vi "Register Sensor View.vi"(11 "Message Enqueuer in":refnum<class "Message Enqueuer.lvclass">) -> (3 "Message Enqueuer out":refnum<class "Message Enqueuer.lvclass">)   [LabVIEW 2013]
uses:
  <vilib>/ActorFramework/Message Enqueuer/Message Enqueuer.lvclass
  <vilib>/ActorFrameworkMVC/View Observer/Registration Message/Registration Message.lvclass
  <vilib>/ActorFrameworkMVC/View Observer/Data Message/Data Message.lvclass
  Models/Sensor Model Messages/Register Sensor Tiles Info Msg/Register Sensor Tiles Info Msg.lvclass
  Models/Sensor Model Messages/Register Sensor Previous Button Visibility Msg/Register Sensor Previous Button Visibility Msg.lvclass
  Models/Sensor Model Messages/Register Sensor Next Button Visibility Msg/Register Sensor Next Button Visibility Msg.lvclass
  Views/Sensor View Messages/Conceret Sensor Tiles Info Msg/Conceret Sensor Tiles Info Msg.lvclass
  Views/Sensor View Messages/Conceret Sensor Previous Button Visibility Msg/Conceret Sensor Previous Button Visibility Msg.lvclass
  Views/Sensor View Messages/Conceret Sensor Next Button Visibility Msg/Conceret Sensor Next Button Visibility Msg.lvclass
  Models/Sensor Model Messages/Register Sensor Move In Previous Msg/Register Sensor Move In Previous Msg.lvclass
  Views/Sensor View Messages/Conceret Move In Previous Msg/Conceret Move In Previous Msg.lvclass
  Models/Sensor Model Messages/Register Sensor Move In Next Msg/Register Sensor Move In Next Msg.lvclass
  Views/Sensor View Messages/Conceret Move In Next Msg/Conceret Move In Next Msg.lvclass
  <vilib>/ActorFrameworkMVC/UI Controller Messages/Subscribe View to Model Msg/Subscribe View to Model Msg.lvclass/Subscribe View to Model Msg.ctl
  <vilib>/ActorFramework/Message Enqueuer/Message Enqueuer.lvclass/Message Enqueuer.ctl
  <vilib>/ActorFramework/Message Enqueuer/Enqueue.vi
  <vilib>/ActorFramework/Message Priority Queue/Priority Enqueue.vi
  <vilib>/ActorFrameworkMVC/UI Controller Messages/Subscribe View to Model Msg/Subscribe View to Model Msg.lvclass
panel:
  out "Array":errorcluster[](array[cluster])
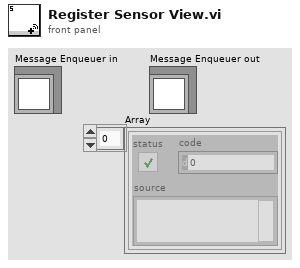
[diagram p1: front panel]
types:
  T1 = cluster{"Registration Message":string, "Data Message":string}[]
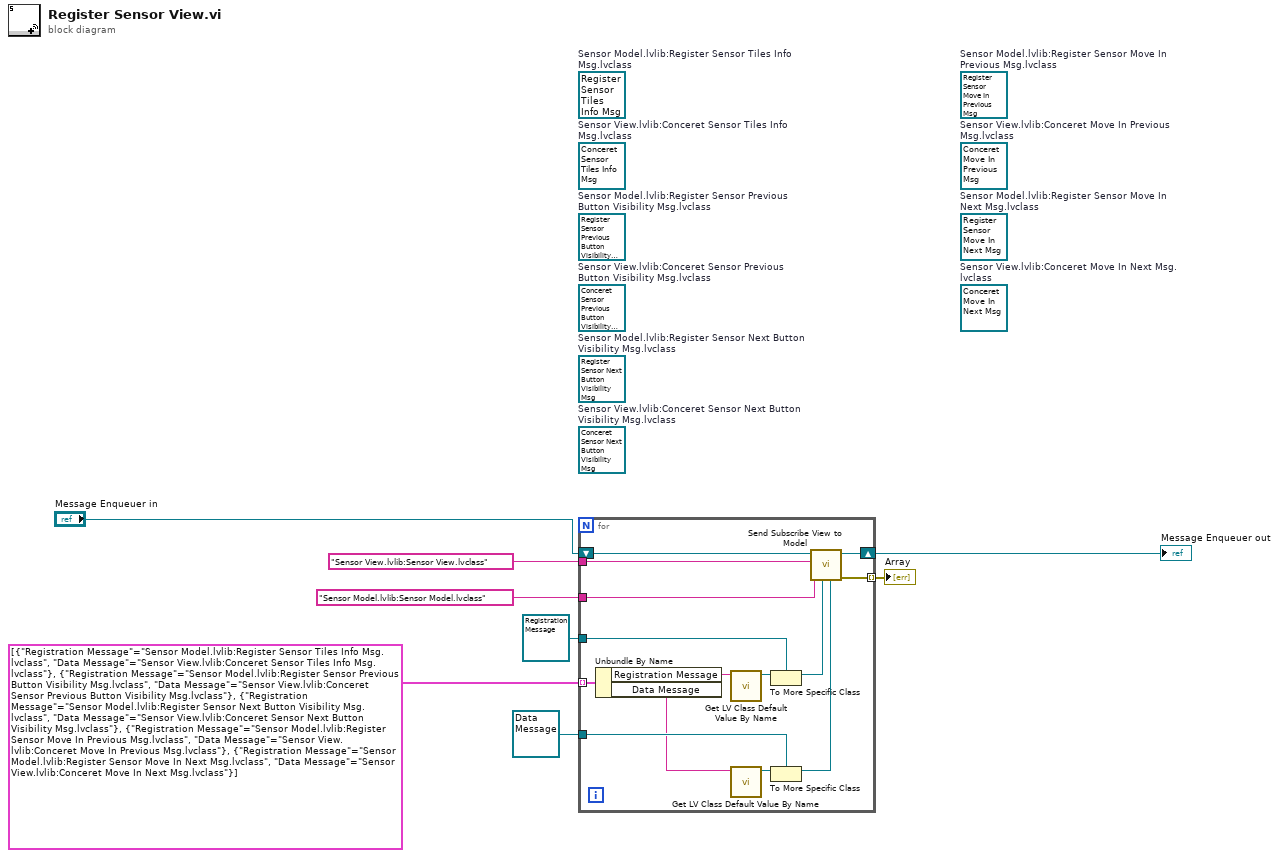
[diagram p0: block diagram]
diagram:
  (unwired) refnum<class "Conceret Move In Next Msg.lvclass"> refnum  # Sensor View.lvlib:Conceret Move In Next Msg.lvclass
  (unwired) refnum<class "Register Sensor Move In Next Msg.lvclass"> refnum  # Sensor Model.lvlib:Register Sensor Move In Next Msg.lvclass
  (unwired) refnum<class "Conceret Move In Previous Msg.lvclass"> refnum  # Sensor View.lvlib:Conceret Move In Previous Msg.lvclass
  (unwired) refnum<class "Register Sensor Move In Previous Msg.lvclass"> refnum  # Sensor Model.lvlib:Register Sensor Move In Previous Msg.lvclass
  (unwired) refnum<class "Conceret Sensor Next Button Visibility Msg.lvclass"> refnum  # Sensor View.lvlib:Conceret Sensor Next Button Visibility Msg.lvclass
  (unwired) refnum<class "Conceret Sensor Previous Button Visibility Msg.lvclass"> refnum  # Sensor View.lvlib:Conceret Sensor Previous Button Visibility Msg.lvclass
  (unwired) refnum<class "Conceret Sensor Tiles Info Msg.lvclass"> refnum  # Sensor View.lvlib:Conceret Sensor Tiles Info Msg.lvclass
  (unwired) refnum<class "Register Sensor Next Button Visibility Msg.lvclass"> refnum  # Sensor Model.lvlib:Register Sensor Next Button Visibility Msg.lvclass
  (unwired) refnum<class "Register Sensor Previous Button Visibility Msg.lvclass"> refnum  # Sensor Model.lvlib:Register Sensor Previous Button Visibility Msg.lvclass
  (unwired) refnum<class "Register Sensor Tiles Info Msg.lvclass"> refnum  # Sensor Model.lvlib:Register Sensor Tiles Info Msg.lvclass
  n1 = for {
    tunnel: "Sensor View.lvlib:Sensor View.lvclass" ("View Name") -> [w21]
    tunnel: "Sensor Model.lvlib:Sensor Model.lvclass" ("Model Name") -> [w20]
    shift-right: [w19] -> w8
    shift-left: "Message Enqueuer in" -> [w22]
    tunnel: refnum<class "Registration Message.lvclass"> refnum ("Registration Message") -> [w16]
    tunnel: refnum<class "Data Message.lvclass"> refnum ("Data Message") -> [w15]
    tunnel: T1 [{"Registration Message"="Sensor Model.lvlib:Register Sensor Tiles Info Msg.lvclass", "Data Message"="Sensor View.lvlib:Conceret Sensor Tiles Info Msg.lvclass"}, {"Registration Message"="Sensor Model.lvlib:Register Sensor Previous Button Visibility Msg.lvclass", "Data Message"="Sensor View.lvlib:Conceret Sensor Previous Button Visibility Msg.lvclass"}, {"Registration Message"="Sensor Model.lvlib:Register Sensor Next Button Visibility Msg.lvclass", "Data Message"="Sensor View.lvlib:Conceret Sensor Next Button Visibility Msg.lvclass"}, {"Registration Message"="Sensor Model.lvlib:Register Sensor Move In Previous Msg.lvclass", "Data Message"="Sensor View.lvlib:Conceret Move In Previous Msg.lvclass"}, {"Registration Message"="Sensor Model.lvlib:Register Sensor Move In Next Msg.lvclass", "Data Message"="Sensor View.lvlib:Conceret Move In Next Msg.lvclass"}] -> [w14] mode=indexing
    tunnel: [w9] -> w1 mode=indexing
    n2 = Unbundle By Name(w14) -> ("Registration Message"=w11:string, "Data Message"=w10:string)
    n3 = call <vilib>:"Get LV Class Default Value By Name.vi"("class name"=w11) -> ("object"=w18:refnum<class>)  [unwired: 9 in, 1 out]
    n4 = call <vilib>:"Get LV Class Default Value By Name.vi"("class name"=w10) -> ("object"=w17:refnum<class>)  [unwired: 9 in, 1 out]
    n5 = To More Specific Class(target class=w16, reference=w18) -> (specific class reference=w13:refnum<class "Registration Message.lvclass">)  [unwired: 1 in, 1 out]
    n6 = To More Specific Class(target class=w15, reference=w17) -> (specific class reference=w12:refnum<class "Data Message.lvclass">)  [unwired: 1 in, 1 out]
    n7 = call <vilib>:"Send Subscribe View to Model.vi"("Data Message"=w12, "Registration Message"=w13, "Model Name"=w20, "View Name"=w21, "Message Enqueuer"=w22) -> ("error out"=w9:errorcluster, "Message Enqueuer out"=w19:refnum<class "Message Enqueuer.lvclass">)  [unwired: 5 in]
  }
  "Message Enqueuer out" <- w8
  "Array" <- w1
